vi "TC Post Build.vi"() -> ()   [LabVIEW 2016]
uses:
  <userlib>/LevyLab/Build Support/PostBuildSupport/PostBuildSupport.lvclass
  <vilib>/MakerHub/Toolbox/LMH-Toolbox.lvlib
panel:
  in  "Package Version":string="4.59.15"
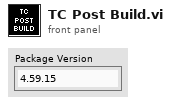
[diagram p1: front panel]
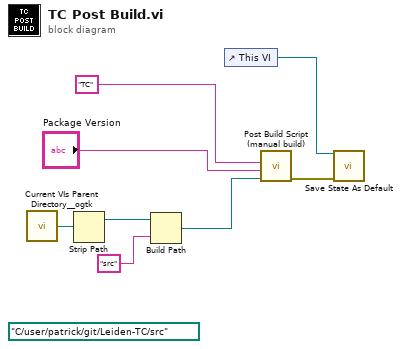
[diagram p0: block diagram]
diagram:
  (unwired) path "C:/user/patrick/git/Leiden-TC/src" ("Package Source Folder")
  n1 = call <userlib>:"Current VIs Parent Directory__ogtk.vi"() -> ("Parent Directory (+ Relative)"=w8:path)  [unwired: 5 in]
  n2 = Strip Path(path=w8) -> (stripped path=w7:path)  [unwired: 1 out]
  n3 = Build Path(base path=w7, name or relative path="src") -> (appended path=w3:path)
  n4 = control-ref of="This VI"() -> (w1:refnum<vi>)
  n5 = call <userlib>:"Post Build Script (manual build).vi"("Package Source Folder"=w3, "Package Version"="Package Version", "Product Name"="TC") -> ("error out"=w2:errorcluster)  [unwired: 8 in]
  n6 = call <vilib>:"Save State As Default.vi"("Error In"=w2, "Target VI"=w1) -> ()  [unwired: 8 in, 2 out]
